vi "CJ switcher().vi"() -> (3 "Guidance Library.lvlib:CJ switcher.lvclass":refnum<class "CJ switcher.lvclass">)   [LabVIEW 2014, in "Guidance Library.lvlib" / "CJ switcher.lvclass"]
uses:
  CJ switcher.lvclass
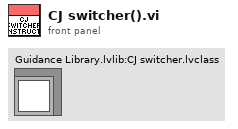
[diagram p1: front panel]
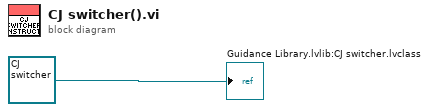
[diagram p0: block diagram]
diagram:
  "Guidance Library.lvlib:CJ switcher.lvclass" <- refnum<class "CJ switcher.lvclass"> refnum ("Guidance Library.lvlib:CJ switcher.lvclass")
